vi "Add VLs and UDPs.vi"(8 "error in (no error)":errorcluster, 10 "VLs":cluster{"VL":u32, "UDP Ports":u32[]}[](array[cluster]), 11 "Section Ref in in":T1 format="%.0x") -> (0 "error out":errorcluster, 3 "Section Ref out":T1 format="%.0x")   [LabVIEW 2020, in "AIM ARINC 664 Scripting.lvlib"]
uses:
  AIM ARINC 664 Scripting.lvlib
  <vilib>/NI VeriStand/Custom Device API/Custom Device Item Ref.ctl
  Constants.vi
  <vilib>/NI VeriStand/Custom Device API/Custom Device API.lvlib
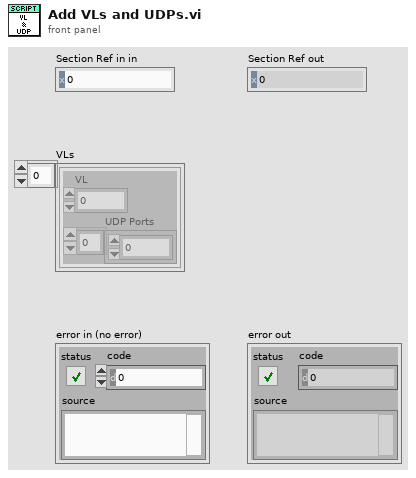
[diagram p1: front panel]
types:
  T1 = typedef "Custom Device API.lvlib/Custom Device Item Ref.ctl" = u64
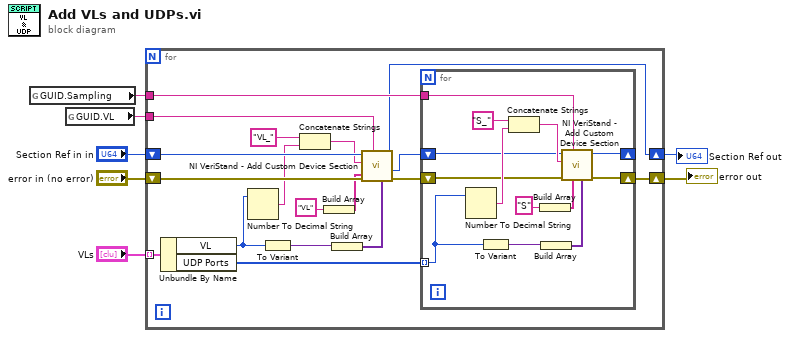
[diagram p0: block diagram]
diagram:
  n1 = global read "Constants.vi" "GUID.Sampling"() -> (w2:string)
  n2 = global read "Constants.vi" "GUID.VL"() -> (w3:string)
  n3 = for {
    tunnel: "VLs" -> [w21] mode=indexing
    shift-right: [w8] -> w1
    shift-left: "Section Ref in in" -> [w25]
    shift-right: [w22] -> w4
    shift-left: "error in (no error)" -> [w24]
    tunnel: w3 -> [w11]
    tunnel: w2 -> [w10]
    n4 = Unbundle By Name(w21) -> ("VL"=w14:u32, "UDP Ports"=w12:u32[])
    n5 = Number To Decimal String(number=w14) -> (decimal integer string=w19:string)  [unwired: 1 in]
    n6 = To Variant(anything=w14) -> (Variant=w13:variant)
    n7 = Concatenate Strings("VL_" ("string"), w19) -> (w18:string)
    n8 = Build Array("VL" ("string")) -> (w17:string[])
    n9 = Build Array(w13) -> (w15:variant[])
    n10 = call <vilib>:"NI VeriStand - Add Custom Device Section.vi"("Property Values"=w15, "Property names"=w17, "GUID (Default Section)"=w11, "error in (no error)"=w24, "Section Name"=w18, "Parent Ref in"=w25) -> ("error out"=w23:errorcluster, "Section Ptr"=w9:T1, "Parent Ref out"=w8:T1)  [unwired: 2 in, 1 out]
    n11 = for {
      shift-right: [w28] -> _
      shift-left: w9 -> [w33]
      shift-right: [w27] -> w22
      shift-left: w23 -> [w32]
      tunnel: w12 -> [w31] mode=indexing
      tunnel: w10 -> [w26]
      n12 = Number To Decimal String(number=w31) -> (decimal integer string=w35:string)  [unwired: 1 in]
      n13 = To Variant(anything=w31) -> (Variant=w30:variant)
      n14 = Concatenate Strings("S_" ("string"), w35) -> (w36:string)
      n15 = Build Array("S" ("string")) -> (w37:string[])
      n16 = Build Array(w30) -> (w29:variant[])
      n17 = call <vilib>:"NI VeriStand - Add Custom Device Section.vi"("Property Values"=w29, "Property names"=w37, "GUID (Default Section)"=w26, "error in (no error)"=w32, "Section Name"=w36, "Parent Ref in"=w33) -> ("error out"=w27:errorcluster, "Parent Ref out"=w28:T1)  [unwired: 2 in, 2 out]
    }
  }
  "Section Ref out" <- w1
  "error out" <- w4
